vi "mod_QAM Lock Detector.vi"(0 "recovered waveform":T2 {"Y" format="%.3f"; "dt" format="%^.2e"; "t0" format="%.4f"}, 5 "QAM system parameters":T1={"samples per symbol (16)"=16, "symbol map"=[]} {"symbol map" format="%.3f"}, 7 "demodulated bit stream":i8[](array[numeric]), 11 "error in (no error)":errorcluster) -> (4 "good lock?":bool, 6 "aggregate\ndecision distance":dbl format="%.2f", 15 "error out":errorcluster)   [LabVIEW 2020, in "niDMT.lvlib"]
uses:
  <vilib>/addons/Modulation/niDMT.lvlib
  <vilib>/addons/Modulation/Analog/controls/Complex Data Waveform.ctl
  <vilib>/addons/Modulation/Digital/Support/Controls/QAM System Parameters.ctl
  <vilib>/addons/Modulation/niAMT.lvlib
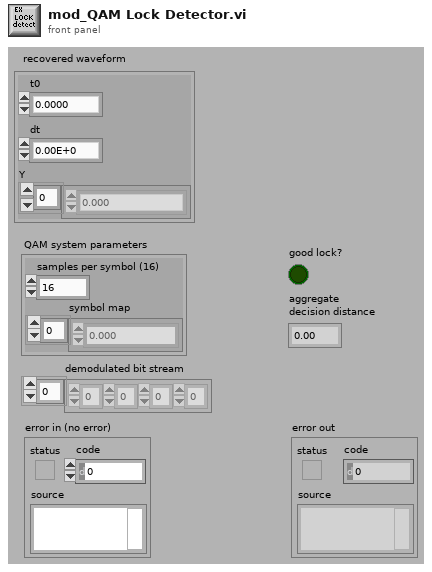
[diagram p1: front panel]
types:
  T1 = typedef "niDMT.lvlib/QAM System Parameters.ctl" = cluster{"samples per symbol (16)":i32, "symbol map":cdb[]}
  T2 = typedef "niAMT.lvlib/Complex Data Waveform.ctl" = cluster{"t0":dbl, "dt":dbl, "Y":cdb[]}
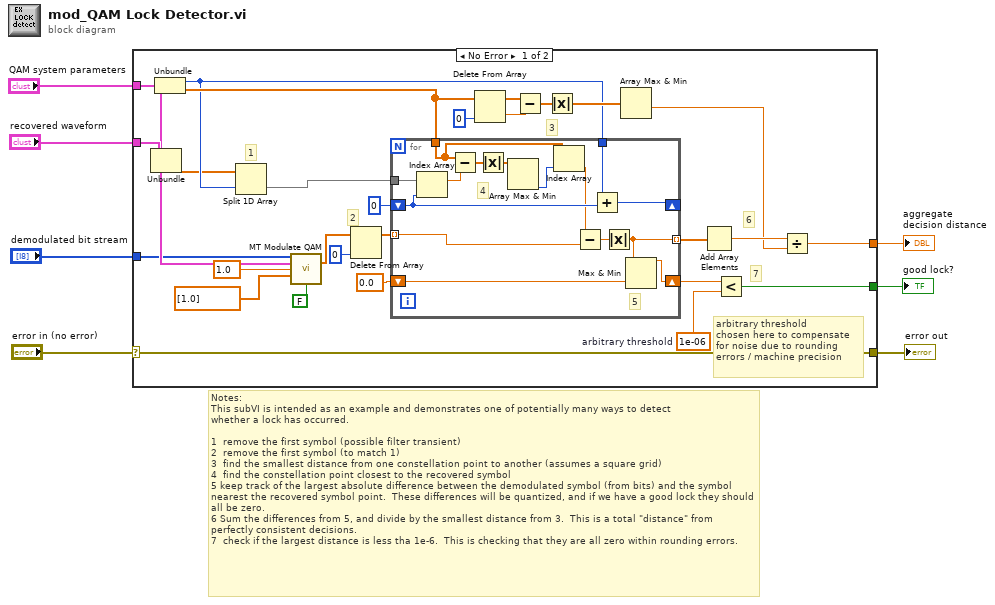
[diagram p0: block diagram]
diagram:
  # "Notes:\nThis subVI is intended as an example and demonstrates one of potentially many ways to detect\nwhether a lock has occurred. \n\n1  remove the first symbol (possible filter transient)\n2  remove the first symbol (to match 1)\n3  find the smallest distance from one constellation point to another (assumes a square grid)\n4  find the constellation point closest to the recovered symbol\n5 keep track of the largest absolute difference between the demodulated symbol (from bits) and the symbol nearest the recovered symbol point.  These differences will be quantized, and if we have a good lock they should all be zero.\n6 Sum the differences from 5, and divide by the smallest distance from 3.  This is a total \"distance\" from perfectly consistent decisions.\n7  check if the largest distance is less tha 1e-6.  This is checking that they are all zero within rounding errors."
  n1 = case shown="No Error" "error in (no error)" {
    selector: "error in (no error)" -> [w24 w51]
    tunnel: "recovered waveform" -> [w35 _]
    tunnel: "QAM system parameters" -> [w34 _]
    tunnel: "demodulated bit stream" -> [w33 _]
    tunnel: [w26 _] -> w4
    tunnel: [w15 _] -> w3
    tunnel: [w24 w51] -> w1
    frame No Error {
      w16 = 1e-06  # arbitrary threshold
      # "arbitrary threshold\nchosen here to compensate\nfor noise due to rounding\nerrors / machine precision"
      # "7"
      # "6"
      # "3"
      # "2"
      # "1"
      n2 = Unbundle(w35) -> ("Y"=w11:cdb[])  [unwired: 2 out]
      n3 = Unbundle(w34) -> ("samples per symbol (16)"=w13:i32, "symbol map"=w23:cdb[])
      n4 = Split 1D Array(array=w11, index=w13) -> (second subarray=w12:cdb[])  [unwired: 1 out]
      n5 = call <vilib>:"MT Modulate QAM.vi"("input bit stream"=w33, "QAM system parameters"=w34, "symbol rate (Hz)"=1.0, "pulse shaping filter coefficients"=dbl[] [1.0], "reset? (T)"=FALSE) -> ("symbols out"=w9:cdb[])  [unwired: 2 in, 8 out]
      n6 = Delete From Array(array=w9, index=0) -> (array with subset deleted=w10:cdb[])  [unwired: 1 in, 1 out]
      n7 = for {
        tunnel: w23 -> [w42]
        tunnel: w10 -> [w40] mode=indexing
        tunnel: w12 -> [w47]
        shift-right: [w50] -> _
        shift-left: 0 -> [w48]
        tunnel: w13 -> [w49]
        shift-right: [w36] -> w27
        shift-left: 0.0 -> [w37]
        tunnel: [w38] -> w17 mode=indexing
        # "5"
        # "4"
        n8 = Index Array(array=w47, index=w48) -> (element=w46:cdb)
        n9 = Subtract(x=w42, y=w46) -> (x-y=w45:cdb[])
        n10 = Absolute Value(x=w45) -> (abs(x)=w44:dbl[])
        n11 = Array Max & Min(array=w44) -> (min index (indices)=w43:i32)  [unwired: 3 out]
        n12 = Index Array(array=w42, index=w43) -> (element=w41:cdb)
        n13 = Subtract(x=w41, y=w40) -> (x-y=w39:cdb)
        n14 = Add(x=w49, y=w48) -> (x+y=w50:i32)
        n15 = Absolute Value(x=w39) -> (abs(x)=w38:dbl)
        n16 = Max & Min(x=w38, y=w37) -> (max(x,y)=w36:dbl)  [unwired: 1 out]
      }
      n17 = Delete From Array(array=w23, index=0) -> (deleted portion=w20:cdb, array with subset deleted=w21:cdb[])  [unwired: 1 in]
      n18 = Subtract(x=w21, y=w20) -> (x-y=w19:cdb[])
      n19 = Absolute Value(x=w19) -> (abs(x)=w18:dbl[])
      n20 = Array Max & Min(array=w18) -> (min value=w14:dbl)  [unwired: 3 out]
      n21 = Add Array Elements(numeric array=w17) -> (sum=w25:dbl)
      n22 = Less?(x=w27, y=w16) -> (x < y?=w26:bool)
      n23 = Divide(x=w25, y=w14) -> (x/y=w15:dbl)
    }
    frame Error {
    }
  }
  "good lock?" <- w4
  "error out" <- w1
  "aggregate\ndecision distance" <- w3
